vi "eraseAI_img.vi"   [LabVIEW 2015]
types:
  T1 = typedef "LVRectTypeDef.ctl" = cluster{"Left":i16, "Top":i16, "Right":i16, "Bottom":i16}
  T2 = cluster{"Xpixels":i32, "Vxminref":dbl, "Vxmaxref":dbl, "P":dbl, "Ypixels":i32, "Vyminref":dbl, "Vymaxref":dbl, "srate":sgl, "sAOxy":i32, "timeout":dbl, "type":string, "date":string, "time":string, "Colormap":u16, "Drawing Mode":u16, "Scanning Mode":u16, "square pixels":bool, "square matrix":bool, "Xpixels Img":i32, "Vx-min Img":dbl, "VX-max Img":dbl, "Ypixels Img":i32, "Vy-min Img":dbl, "Vy-max Img ":dbl, "Angle Img":dbl, "autoshutter":bool, "finite":bool, "cont":bool, "wavdet":bool, "measpoints":i32, "avpp":i32, "bufferAO":i32, "bufferAI":i32, "starttick":u32, "waveform":path, "Vx-ref":dbl, "Vy-ref":dbl, "refreshrate":dbl, "refreshbuffer":i32, "tt_cycles":i32, "motorref":refnum<k7>, "mirrorswitch":refnum<k7>, "sample mode":i32, "maxbufferAI":i32, "srateAODO":sgl, "bin":sgl, "Pel":sgl, "Angle draw":dbl, "srate Img":sgl, "ROIimg_plotbounds":T1, "auto OD":bool, "ODfilt":u16, "aAI":i32[], "aCI":i32[], "aAO":u32[], "aDO":u32[], "refwfsize":dbl, "Lifetime":bool, "Vz-Img":dbl, "Vz-ref":dbl, "Vz-reset":dbl, "AIoverride":bool}
  T3 = cluster{" AI":refnum<k21>, "E_AI":errorcluster, "header":dbl[]}
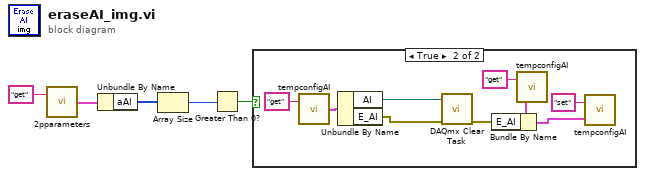
[diagram p0: block diagram]
diagram:
  n1 = call "2pparameters.vi"("command"="get") -> ("params out"=w4:T2)  [unwired: 1 in]
  n2 = Unbundle By Name(w4) -> ("aAI"=w3:i32[])
  n3 = Array Size(array=w3) -> (size(s)=w2:i32)
  n4 = Greater Than 0?(x=w2) -> (x > 0?=w1:bool)
  n5 = case shown="True" w1 {
    frame False {
    }
    frame True {
      n6 = call "tempconfigAI.vi"("command"="get") -> ("Temp Config out"=w12:T3)  [unwired: 1 in]
      n7 = Unbundle By Name(w12) -> ("AI"=w7:refnum<k21>, "E_AI"=w6:errorcluster)
      n8 = call <vilib>:"DAQmx Clear Task.vi"("task in"=w7, "error in"=w6) -> ("error out"=w9:errorcluster)  [unwired: 13 in]
      n9 = call "tempconfigAI.vi"("command"="get") -> ("Temp Config out"=w14:T3)  [unwired: 1 in]
      n10 = Bundle By Name(cluster=w14, "E_AI"=w9) -> (w8:T3)
      n11 = call "tempconfigAI.vi"("Temp Config in"=w8, "command"="set") -> ()  [unwired: 1 out]
    }
  }
